vi "WPI_DashboardManage Camera Display Indices.vi"(8 "Operation":enum16{"Add", "Retrieve"}(ring)=enum."Retrieve", 11 "Display Name":string) -> (3 "index of element":i32)   [LabVIEW 2025]
uses:
  <vilib>/Rock Robotics/WPI/Dashboard/WPI_DashboardLogging Global.vi
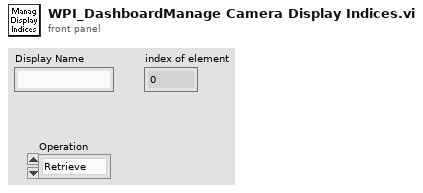
[diagram p1: front panel]
types:
  T1 = cluster{"Video 1":i32, "Video 2":i32, "Video 3":i32, "Video 4":i32}
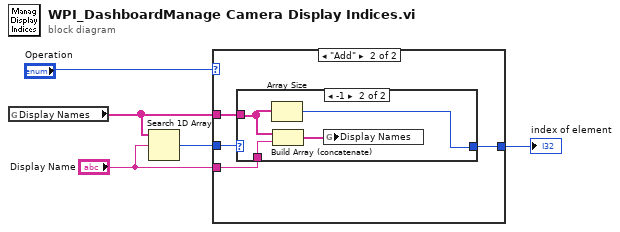
[diagram p0: block diagram]
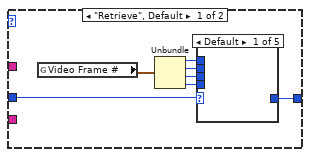
[diagram p2: hidden frame]
diagram:
  n1 = global read "WPI_DashboardLogging Global.vi" "Display Names"() -> (w3:string[])
  n2 = Search 1D Array(1D array=w3, element="Display Name") -> (index of element=w2:i32)  [unwired: 1 in]
  n3 = case shown="\"Add\"" "Operation" {
    tunnel: [w10 w20] -> w5
    tunnel: "Display Name" -> [_ w19]
    tunnel: w3 -> [_ w18]
    tunnel: w2 -> [w11 w17]
    frame "Retrieve", Default {
      n4 = global read "WPI_DashboardLogging Global.vi" "Video Frame #"() -> (w12:T1)
      n5 = Unbundle(w12) -> ("Video 1"=w9:i32, "Video 2"=w8:i32, "Video 3"=w7:i32, "Video 4"=w6:i32)
      n6 = case shown="Default" w11 {
        tunnel: [_ w13 w14 w15 w16] -> w10
        tunnel: w9 -> [_ w13 _ _ _]
        tunnel: w8 -> [_ _ w14 _ _]
        tunnel: w7 -> [_ _ _ w15 _]
        tunnel: w6 -> [_ _ _ _ w16]
        frame Default {
        }
        frame 0 {
        }
        frame 1 {
        }
        frame 2 {
        }
        frame 3 {
        }
      }
    }
    frame "Add" {
      n7 = case shown="-1" w17 {
        selector: w17 -> [w21 _]
        tunnel: [w21 w22] -> w20
        tunnel: w18 -> [_ w25]
        tunnel: w19 -> [_ w24]
        frame Default {
        }
        frame -1 {
          n8 = Array Size(array=w25) -> (size(s)=w22:i32)
          n9 = Build Array (concatenate)(w25, w24) -> (w23:string[])
          n10 = global write "WPI_DashboardLogging Global.vi" "Display Names"(w23) -> ()
        }
      }
    }
  }
  "index of element" <- w5
